vi "Destroy Lookup Table.vi"(8 "error in (no error)":errorcluster, 11 "LookupTable Reference":refnum<data-value>) -> (0 "error out":errorcluster)   [LabVIEW 2017, in "LookupTable.lvlib" / "LookupTable.lvclass"]
uses:
  <vilib>/gpm_packages/@cs/lookup-table/Source/LookupTable/LookupTable.lvclass
  <vilib>/gpm_packages/@cs/lookup-table/Source/LookupTable/LookupTable.lvclass/LookupTable.ctl
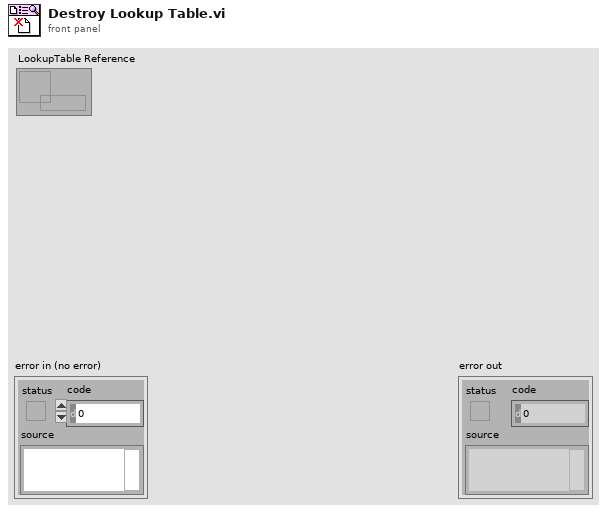
[diagram p1: front panel]
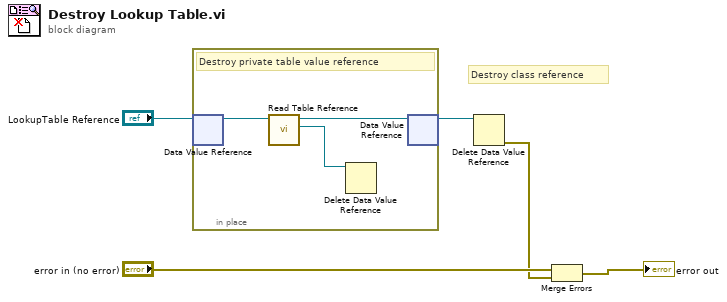
[diagram p0: block diagram]
diagram:
  # "Destroy class reference"
  n1 = in-place {
    # "Destroy private table value reference"
    n2 = in-place-dvr #1("LookupTable Reference") -> (w8:refnum<class "LookupTable.lvclass">)  [unwired: 1 out]
    n3 = call <vilib>:"Read Table Reference.vi"("LookupTable in"=w8) -> ("Table Reference"=w7:refnum<data-value>, "LookupTable out"=w6:refnum<class "LookupTable.lvclass">)  [unwired: 9 in]
    n4 = Delete Data Value Reference(data value reference=w7) -> ()  [unwired: 1 in, 2 out]
    n5 = in-place-dvr #1(w6) -> (w2:refnum<data-value>)  [unwired: 1 out]
  }
  n6 = Delete Data Value Reference(data value reference=w2) -> (error out=w1:errorcluster)  [unwired: 1 in, 1 out]
  n7 = Merge Errors("error in (no error)", w1) -> (→"error out":errorcluster)
